vi "Template - Function Generator Standard Waveform.vi"() -> ()   [LabVIEW 2011]
doc: "This example shows how to generate a standard waveform."
uses:
  <instrlib>/_Template - Function Generator/Template - Function Generator.lvlib
panel:
  in  "Serial Configuration":T1={"Baud Rate"=9600, "Parity"=0, "Data Bits"=7, "Stop Bits"=10, "Flow Control"=0} {"Flow Control" items=["None", "XON/XOFF", "RTS/CTS", "XON/XOFF & RTS/CTS", "DTR/DSR", "XON/XOFF & DTR/DSR"]; "Stop Bits" items=["1.0"=10, "1.5"=15, "2.0"=20]; "Data Bits" items=["7"=7, "8"=8]; "Parity" items=["None", "Odd", "Even", "Mark", "Space"]; "Baud Rate" items=["300"=300, "600"=600, "1200"=1200, "2400"=2400, "4800"=4800, "9600"=9600, "19200"=19200]}
  in  "DC Offset (0.00 V)":dbl
  in  "Frequency (1000 Hz)":dbl=1000.0
  in  "Amplitude (0.1 Vpp)":dbl=0.1
  in  "Waveform Function (0: Sine)":u16(ring) items=["Sine", "Square", "Triangle"]
  in  "VISA resource name":refnum<visa-resource-name>
  # "(c) 2007 <Enter Company Name Here>.  ALL RIGHTS RESERVED."
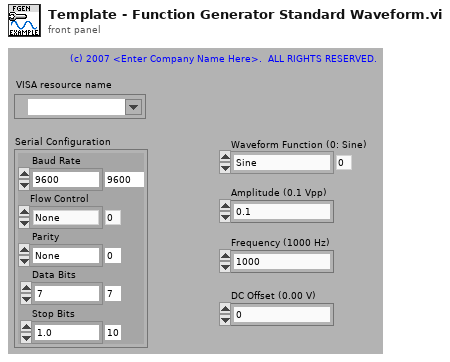
[diagram p1: front panel]
types:
  T1 = cluster{"Baud Rate":u32, "Parity":u16, "Data Bits":u16, "Stop Bits":u16, "Flow Control":u16}
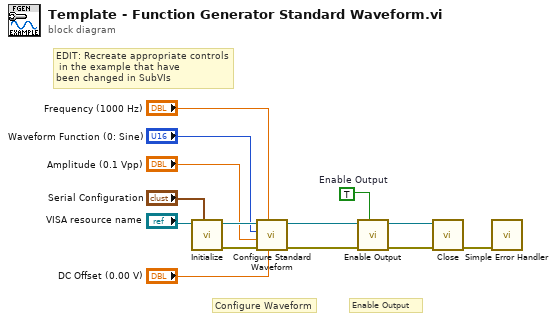
[diagram p0: block diagram]
diagram:
  w1 = TRUE  # Enable Output
  # "EDIT: Recreate appropriate controls\n in the example that have \nbeen changed in SubVIs"
  # "Enable Output"
  # "Configure Waveform"
  n1 = call <instrlib>:"Initialize.vi"("Serial Configuration"="Serial Configuration", "VISA resource name"="VISA resource name") -> ("error out"=w12:errorcluster, "VISA resource name out"=w13:refnum<visa-resource-name>)  [unwired: 8 in]
  n2 = call <instrlib>:"Configure Standard Waveform.vi"("DC Offset (0.00 V)"="DC Offset (0.00 V)", "Frequency (1000 Hz)"="Frequency (1000 Hz)", "error in (no error)"=w12, "Amplitude (1.0 Vpp)"="Amplitude (0.1 Vpp)", "Waveform Function (0: Sine)"="Waveform Function (0: Sine)", "VISA resource name"=w13) -> ("error out"=w7:errorcluster, "VISA resource name out"=w8:refnum<visa-resource-name>)  [unwired: 4 in]
  n3 = call <instrlib>:"Enable Output.vi"("Enable Output (T: Enable)"=w1, "error in (no error)"=w7, "VISA resource name"=w8) -> ("error out"=w5:errorcluster, "VISA resource name out"=w6:refnum<visa-resource-name>)  [unwired: 7 in]
  n4 = call <instrlib>:"Close.vi"("error in (no error)"=w5, "VISA resource name"=w6) -> ("error out"=w9:errorcluster)  [unwired: 9 in]
  n5 = call <vilib>:"Simple Error Handler.vi"("error in (no error)"=w9) -> ()  [unwired: 4 in, 5 out]
